vi "Ini files Objects.vi"() -> ()   [LabVIEW 2019]
uses:
  Classes/Parse/ParsePaths/Path.lvclass
  Classes/Parse/Dot/Dot.lvclass
  Classes/Parse/Image/SVGImage.lvclass
  Classes/Parse/Rectangle/Rectangle.lvclass
  Classes/Settings/Dot Settings/Dot Settings.lvclass
  Classes/Settings/Setting Database/Typedefs/PublicEvents--Setting Database.DotsUpdated.ctl
  Classes/Settings/Setting Database/Setting Database.lvclass
  Classes/Settings/Funnel Settings/Funnel Settings.lvclass
  Classes/Settings/Setting Database/Typedefs/PublicEvents--Setting Database.FunnelsUpdated.ctl
  Classes/Settings/Rectangle Settings/Rectangle Settings.lvclass
  Classes/Settings/Setting Database/Typedefs/PublicEvents--Setting Database.RectanglesUpdated.ctl
  Classes/Settings/Path Settings/Path Settings.lvclass
  Classes/Settings/Setting Database/Typedefs/PublicEvents--Setting Database.PathsUpdated.ctl
  Classes/Parse/PathCommands.Moveto/PathCommands.MoveTo.lvclass
  Classes/Parse/PathCommands.CurveTo/PathCommands.CurveTo.lvclass
  Classes/Parse/CSSProperties/CSSProperties.lvclass
  Classes/Parse/Transform.Translate/Transform.Translate.lvclass
  Classes/Parse/PathCommands.LineTo/PathCommands.LineTo.lvclass
  Classes/Parse/Transform.Matrix/Transform.Matrix.lvclass
  Classes/Parse/PathCommands.ClosePath/PathCommands.ClosePath.lvclass
  <vilib>/JKI/JKI SMO/SMO/SMO.lvclass
  <vilib>/JKI/JKI SMO/SMO/Typedefs/SMOState --Enum.ctl
  Classes/Settings/Setting Database/Typedefs/PrivateEvents--Setting Database.Refresh.ctl
  Classes/Archiver/Archivist.lvclass
  <userlib>/_OpenG.lib/lvzip/lvzip.llb/subVI/ZLIB Compress Directory (Path)__ogtk.vi
  C:/Users/Albro/Documents/GitHub/AFM-Lithography/lvsrc/Classes/Settings/ObjectSettings/ObjectSettings.lvclass
  C:/Program Files (x86)/National Instruments/LabVIEW 2019/vi.lib/JKI/JKI SMO/SMO/SMO.lvclass
panel:
  out "GUIDs 2":string[](array[string])
  out "GUIDs":string[](array[string])
  out "Funnels All Updated":bool
  out "Funnels Equal":bool
  out "Rects Equal?":bool
  out "Paths Equal":bool
  out "number of events discarded":u32
  out "Rectangles All Updated":bool
  out "Paths Updated/":bool
  out "error out":errorcluster
  out "Array":string[](array[string])
  out "GUID":string[](array[string])
  # "Why arent GUIDs in Order?"
  # "Close Panel to stop the SMO\n(press the \"X\")"
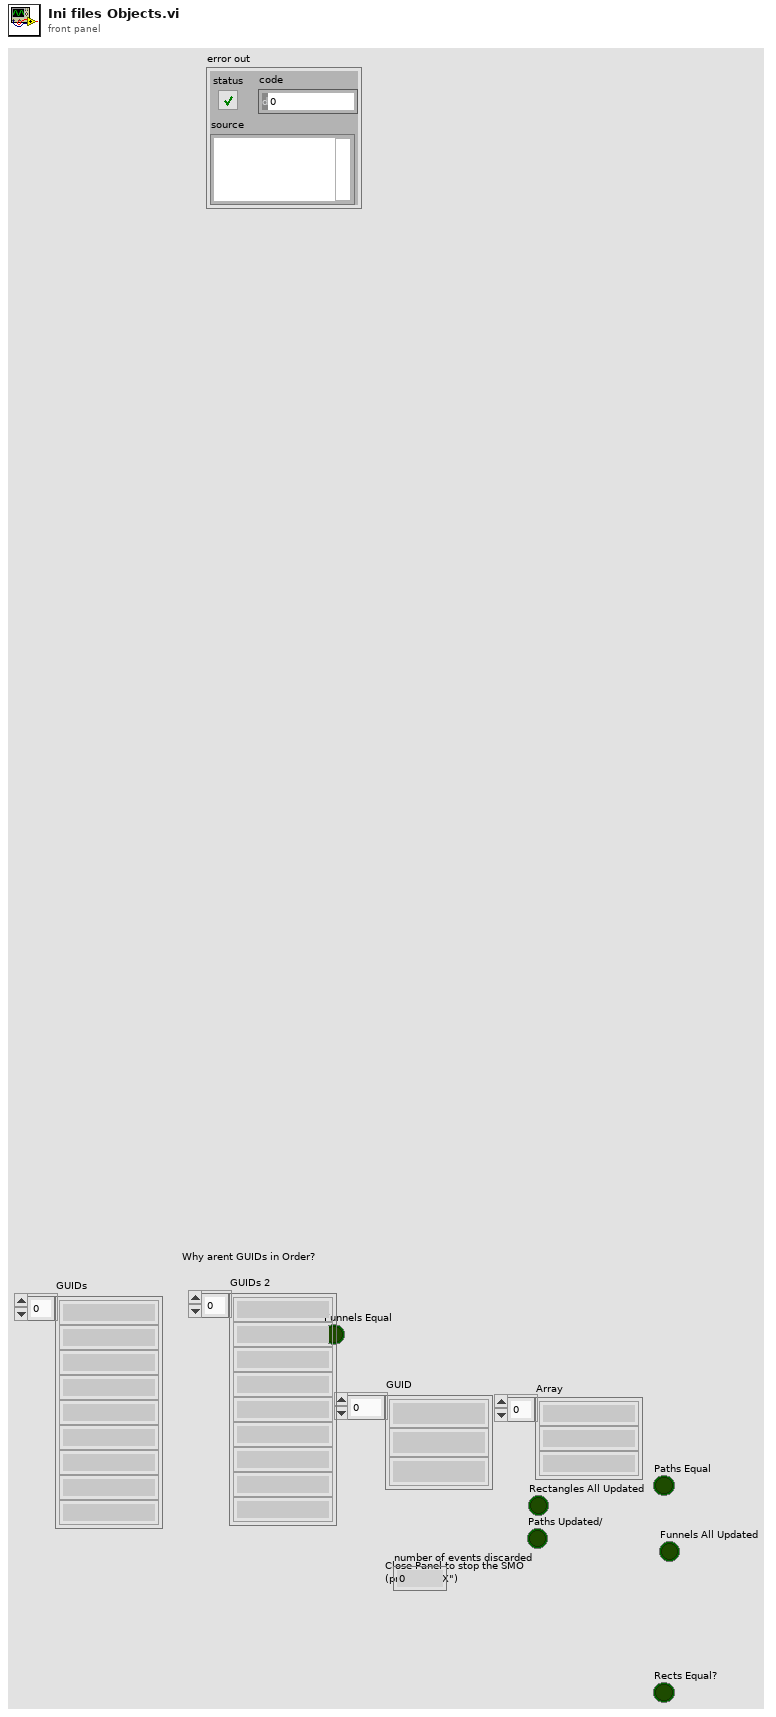
[diagram p1: front panel]
types:
  T1 = typedef "Setting Database.lvclass/PublicEvents--Setting Database.PathsUpdated.ctl" = refnum<class "Path Settings.lvclass">[]
  T2 = typedef "Setting Database.lvclass/PublicEvents--Setting Database.RectanglesUpdated.ctl" = refnum<class "Rectangle Settings.lvclass">[]
  T3 = typedef "Setting Database.lvclass/PublicEvents--Setting Database.FunnelsUpdated.ctl" = refnum<class "Funnel Settings.lvclass">[]
  T4 = typedef "Setting Database.lvclass/PublicEvents--Setting Database.DotsUpdated.ctl" = refnum<class "Dot Settings.lvclass">[]
  T5 = cluster{"Paths":T1, "Rectangles":T2, "Funnels":T3, "Dots":T4}
  T6 = typedef "Setting Database.lvclass/PublicEvents--Cluster.ctl" = cluster{"NewActivePath":refnum<user-event>, "PathsUpdated":refnum<user-event>, "RectanglesUpdated":refnum<user-event>, "NewActiveRectangle":refnum<user-event>, "NewActiveFunnel":refnum<user-event>, "FunnelsUpdated":refnum<user-event>, "NewActiveDot":refnum<user-event>, "DotsUpdated":refnum<user-event>}
  T7 = typedef "SMO.lvclass/Public Events.ctl" = cluster{"Error":refnum<user-event>, "State":refnum<user-event>, "Reserve State":refnum<user-event>}
  T8 = cluster{"Event Registration Refnum":refnum<event-registration>}
  T9 = typedef "Setting Database.lvclass/PrivateEvents--Setting Database.Refresh.ctl" = cluster{"Paths":string[], "Rectangles":string[], "Funnels":string[], "Dots":string[]}
  T10 = cluster{"Settings":cluster{"Paths":T1, "Rectangles":T2, "Funnels":T3, "Dots":T4}, "Data":cluster{"Paths":refnum<class "Path.lvclass">[], "Rectangles":refnum<class "Rectangle.lvclass">[], "SVGImage":refnum<class "SVGImage.lvclass">, "Dots":refnum<class "Dot.lvclass">[], "Funnels":refnum<class "Path.lvclass">[]}}
  T11 = cluster{"paths":string[], "funnels":string[], "rects":string[], "dots":string[]}
  T12 = enum16{"open", "replace", "create", "open or create", "replace or create", "replace or create with confirmation"}
  T13 = typedef "SMO.lvclass/SMOState --Enum.ctl" = enum16{"unknown", "Created", "Started", "Stopped"}
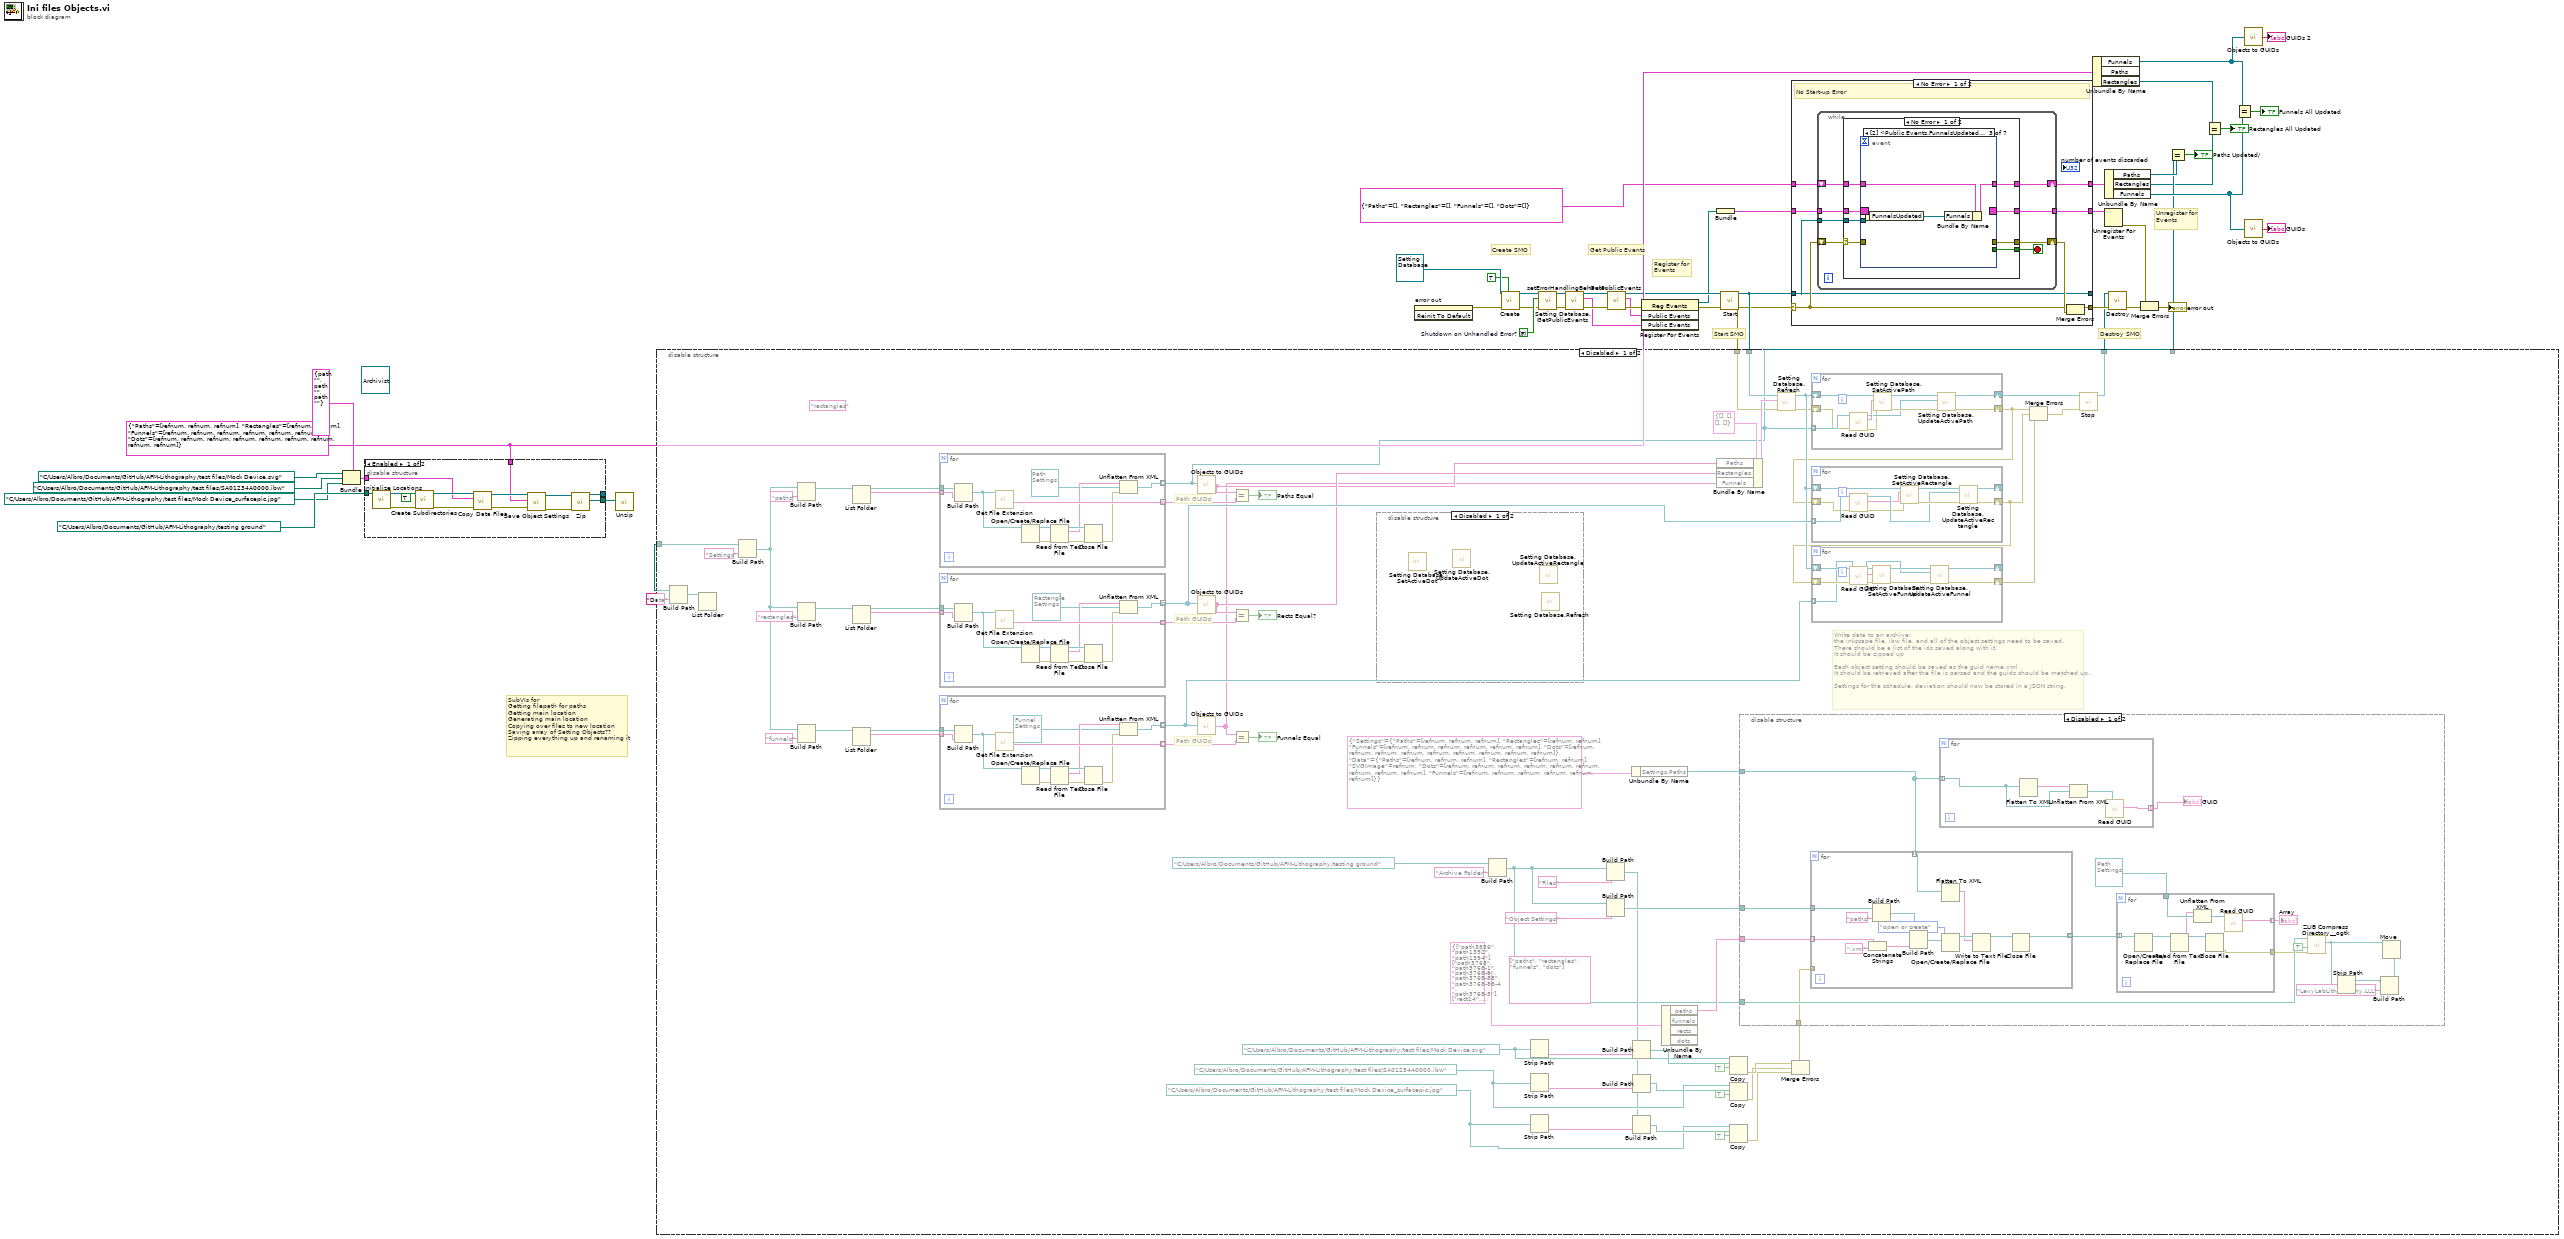
[diagram p0: block diagram]
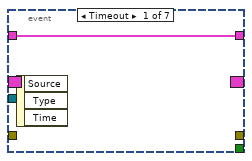
[diagram p2: hidden frame]
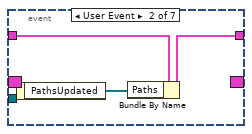
[diagram p3: hidden frame]
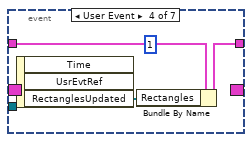
[diagram p4: hidden frame]
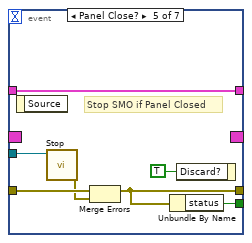
[diagram p5: hidden frame]
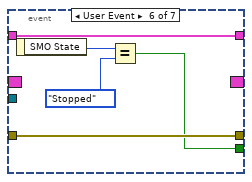
[diagram p6: hidden frame]
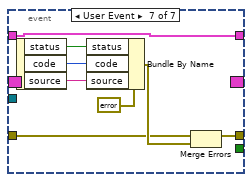
[diagram p7: hidden frame]
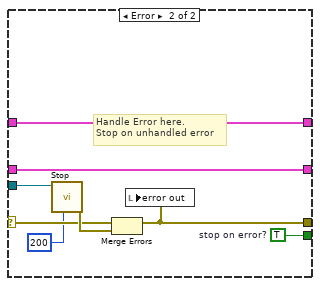
[diagram p8: hidden frame]
diagram:
  w37 = TRUE  # Shutdown on Unhandled Error? (F)
  (unwired) refnum<class "Archivist.lvclass"> refnum ("Archivist.lvclass")
  w42 = T5 {"Paths"=[refnum, refnum, refnum], "Rectangles"=[refnum, refnum], "Funnels"=[refnum, refnum, refnum, refnum, refnum, refnum], "Dots"=[refnum, refnum, refnum, refnum, refnum, refnum, refnum, refnum, refnum]} ("Settings")
  # "Get Public Events"
  # "Start SMO"
  # "Destroy SMO"
  # "Create SMO"
  # "Unregister for Events"
  # "Register for Events"
  # "SubVIs for \nGetting filepath for paths\nGetting main location\nGenerating main location\nCopying over files to new location\nSaving array of Setting Objects??\nZipping everything up and renaming it"
  n1 = Bundle(cluster=cluster{"svg":path, "afm":path, "jpg":path} {"svg"=path "", "afm"=path "", "jpg"=path ""}, "svg"=path "C:/Users/Albro/Documents/GitHub/AFM-Lithography/test files/Mock Device.svg" ("file path"), "afm"=path "C:/Users/Albro/Documents/GitHub/AFM-Lithography/test files/SA01234A0000.ibw" ("file path"), "jpg"=path "C:/Users/Albro/Documents/GitHub/AFM-Lithography/test files/Mock Device_surfacepic.jpg" ("file path")) -> (w41:cluster{"svg":path, "afm":path, "jpg":path})
  n2 = disable-structure shown="Enabled" {
    disable-tunnel: path "C:/Users/Albro/Documents/GitHub/AFM-Lithography/testing ground" ("file path") -> [w60 _]
    disable-tunnel: w42 -> [w56 _]
    disable-tunnel: w41 -> [w55 _]
    disable-tunnel: [w49 _] -> w40
    disable-tunnel: [w48 _] -> _
    frame Enabled {
      (unwired) TRUE ("Archive?")
      n3 = call "Initialize Locations.vi"("Save Location"=w60) -> ("error out"=w54:errorcluster, "Archivist out"=w59:refnum<class "Archivist.lvclass">)  [unwired: 9 in]
      n4 = call "Create Subdirectories.vi"("error in"=w54, "Archivist in"=w59) -> ("error out"=w53:errorcluster, "Archivist out"=w58:refnum<class "Archivist.lvclass">)  [unwired: 8 in]
      n5 = call "Copy Data Files.vi"("error in"=w53, "Data Files"=w55, "Archivist in"=w58) -> ("error out"=w52:errorcluster, "Archivist out"=w57:refnum<class "Archivist.lvclass">)  [unwired: 7 in]
      n6 = call "Save Object Settings.vi"("error in"=w52, "Settings"=w56, "Archivist in"=w57) -> ("error out"=w50:errorcluster, "Archivist out"=w51:refnum<class "Archivist.lvclass">)  [unwired: 7 in]
      n7 = call "Zip.vi"("error in"=w50, "Archivist in"=w51) -> ("archive name out"=w49:path, "Archivist out"=w48:refnum<class "Archivist.lvclass">)  [unwired: 7 in, 1 out]
    }
    frame Disabled {
    }
  }
  n8 = call "Unzip.vi"("Path"=w40) -> ()  [unwired: 9 in, 2 out]
  n9 = invoke on="error out" class="Clust (strict)" method="Reinit To Default"() -> (error out=w38:errorcluster)  [unwired: 3 in, 2 out]
  n10 = call <vilib>:"Create.vi"("Shared Resource (F)"=TRUE, "error in (no error)"=w38, "SMO"=refnum<class "Setting Database.lvclass"> refnum ("Setting Database.lvclass")) -> ("error out"=w36:errorcluster, "SMO out"=w35:refnum<class "Setting Database.lvclass">)  [unwired: 6 in, 1 out]
  n11 = call <vilib>:"setErrorHandlingBehavior.vi"("error in (no error)"=w36, "Shutdown on Unhandled Error? (F)"=w37, "SMO in"=w35) -> ("error out"=w20:errorcluster, "SMO out"=w22:refnum<class "Setting Database.lvclass">)  [unwired: 7 in]
  n12 = call "Setting Database.GetPublicEvents.vi"("error in (no error)"=w20, "Setting Database"=w22) -> ("error out"=w19:errorcluster, "Public Events"=w18:T6, "Setting Database out"=w21:refnum<class "Setting Database.lvclass">)  [unwired: 7 in]
  n13 = call <vilib>:"GetPublicEvents.vi"("error in (no error)"=w19, "SMO"=w21) -> ("error out"=w33:errorcluster, "Public Events"=w32:T7, "SMO out"=w39:refnum<class "Setting Database.lvclass">)  [unwired: 7 in]
  n14 = register-events(error in=w33, w32, w18) -> (reference out=w30:refnum<event-registration>, error out=w31:errorcluster)  [unwired: 1 in]
  n15 = Bundle("Event Registration Refnum"=w30) -> (w26:T8)  [unwired: 1 in]
  n16 = call <vilib>:"Start.vi"("error in (no error)"=w31, "SMO"=w39) -> ("error out"=w11:errorcluster, "SMO out"=w12:refnum<class "Setting Database.lvclass">)  [unwired: 8 in]
  n17 = disable-structure shown="Disabled" {
    disable-tunnel: [w101 _] -> w17
    disable-tunnel: w12 -> [w97 _]
    disable-tunnel: w11 -> [w96 _]
    disable-tunnel: [w62 _] -> w4
    disable-tunnel: [w61 _] -> w1
    frame Disabled {
      (unwired) "rectangles" ("pattern")
      w107 = path "C:/Users/Albro/Documents/GitHub/AFM-Lithography/test files/Mock Device_surfacepic.jpg" ("file path")
      w113 = path "C:/Users/Albro/Documents/GitHub/AFM-Lithography/test files/SA01234A0000.ibw" ("file path")
      w117 = path "C:/Users/Albro/Documents/GitHub/AFM-Lithography/test files/Mock Device.svg" ("file path")
      (unwired) string[] ["paths", "rectangles", "funnels", "dots"]
      # "Path GUIDs"
      # "Path GUIDs"
      # "Path GUIDs"
      # "Write data to an archive:\nthe inkscape file, ibw file, and all of the object settings need to be saved. \nThere should be a list of the ids saved along with it.\nIt should be zipped up\n\nEach object setting should be saved as the guid name.xml\nIt should be retrieved after the file is parsed and the guids should be matched up..\n\nSettings for the schedule, deviation should now be stored in a JSON string."
      n18 = Build Path(base path=w61, name or relative path="Data") -> (appended path=w92:path)
      n19 = List Folder(path=w92) -> ()  [unwired: 3 in, 4 out]
      n20 = Build Path(base path=w61, name or relative path="Settings") -> (appended path=w73:path)
      n21 = Build Path(base path=w73, name or relative path="paths") -> (appended path=w88:path)
      n22 = Build Path(base path=w73, name or relative path="rectangles") -> (appended path=w83:path)
      n23 = Build Path(base path=w73, name or relative path="funnels") -> (appended path=w77:path)
      n24 = List Folder(path=w88) -> (path out=w87:path, filenames=w86:string[])  [unwired: 3 in, 2 out]
      n25 = List Folder(path=w83) -> (path out=w84:path, filenames=w85:string[])  [unwired: 3 in, 2 out]
      n26 = List Folder(path=w77) -> (path out=w78:path, filenames=w79:string[])  [unwired: 3 in, 2 out]
      n27 = for {
        tunnel: w86 -> [w172] mode=indexing
        tunnel: w87 -> [w173]
        tunnel: [w171] -> w90 mode=indexing
        tunnel: [w163] -> w62 mode=indexing
        n28 = Build Path(base path=w173, name or relative path=w172) -> (appended path=w170:path)
        n29 = call <vilib>:"Get File Extension.vi"("file"=w170) -> ("filename without extension"=w171:string)  [unwired: 6 in, 4 out]
        n30 = Open/Create/Replace File(file path (use dialog)=w170) -> (refnum out=w169:refnum<file>, error out=w167:errorcluster)  [unwired: 5 in, 1 out]
        n31 = Read from Text File(file (use dialog)=w169, error in=w167) -> (refnum out=w168:refnum<file>, text=w165:string, error out=w166:errorcluster)  [unwired: 2 in, 1 out]
        n32 = Close File(refnum=w168, error in=w166) -> (error out=w162:errorcluster)  [unwired: 1 out]
        n33 = Unflatten From XML(xml string=w165, type=refnum<class "Path Settings.lvclass"> refnum ("Path Settings.lvclass"), error in (no error)=w162) -> (value=w163:refnum<class "Path Settings.lvclass">)  [unwired: 1 out]
      }
      n34 = for {
        tunnel: w85 -> [w160] mode=indexing
        tunnel: w84 -> [w161]
        tunnel: [w159] -> w81 mode=indexing
        tunnel: [w152] -> w72 mode=indexing
        n35 = Build Path(base path=w161, name or relative path=w160) -> (appended path=w158:path)
        n36 = call <vilib>:"Get File Extension.vi"("file"=w158) -> ("filename without extension"=w159:string)  [unwired: 6 in, 4 out]
        n37 = Open/Create/Replace File(file path (use dialog)=w158) -> (refnum out=w157:refnum<file>, error out=w155:errorcluster)  [unwired: 5 in, 1 out]
        n38 = Read from Text File(file (use dialog)=w157, error in=w155) -> (refnum out=w156:refnum<file>, text=w153:string, error out=w154:errorcluster)  [unwired: 2 in, 1 out]
        n39 = Close File(refnum=w156, error in=w154) -> (error out=w151:errorcluster)  [unwired: 1 out]
        n40 = Unflatten From XML(xml string=w153, type=refnum<class "Rectangle Settings.lvclass"> refnum ("Rectangle Settings.lvclass"), error in (no error)=w151) -> (value=w152:refnum<class "Rectangle Settings.lvclass">)  [unwired: 1 out]
      }
      n41 = for {
        tunnel: w79 -> [w148] mode=indexing
        tunnel: w78 -> [w149]
        tunnel: [w147] -> w75 mode=indexing
        tunnel: [w140] -> w69 mode=indexing
        n42 = Build Path(base path=w149, name or relative path=w148) -> (appended path=w146:path)
        n43 = call <vilib>:"Get File Extension.vi"("file"=w146) -> ("filename without extension"=w147:string)  [unwired: 6 in, 4 out]
        n44 = Open/Create/Replace File(file path (use dialog)=w146) -> (refnum out=w145:refnum<file>, error out=w143:errorcluster)  [unwired: 5 in, 1 out]
        n45 = Read from Text File(file (use dialog)=w145, error in=w143) -> (refnum out=w144:refnum<file>, text=w141:string, error out=w142:errorcluster)  [unwired: 2 in, 1 out]
        n46 = Close File(refnum=w144, error in=w142) -> (error out=w139:errorcluster)  [unwired: 1 out]
        n47 = Unflatten From XML(xml string=w141, type=refnum<class "Funnel Settings.lvclass"> refnum ("Funnel Settings.lvclass"), error in (no error)=w139) -> (value=w140:refnum<class "Funnel Settings.lvclass">)  [unwired: 1 out]
      }
      n48 = call "Objects to GUIDs.vi"("Objects"=w62) -> ("GUIDs"=w70:string[])  [unwired: 3 in, 1 out]
      n49 = call "Objects to GUIDs.vi"("Objects"=w72) -> ("GUIDs"=w71:string[])  [unwired: 3 in, 1 out]
      n50 = call "Objects to GUIDs.vi"("Objects"=w69) -> ("GUIDs"=w68:string[])  [unwired: 3 in, 1 out]
      n51 = Equal?(x=w70, y=w90) -> (x = y?=→"Paths Equal":bool)
      n52 = Equal?(x=w71, y=w81) -> (x = y?=→"Rects Equal?":bool)
      n53 = Equal?(x=w68, y=w75) -> (x = y?=→"Funnels Equal":bool)
      n54 = disable-structure shown="Disabled" {
        frame Disabled {
          n55 = call "Setting Database.SetActiveDot.vi"() -> ()  [unwired: 10 in, 2 out]
          n56 = call "Setting Database.UpdateActiveDot.vi"() -> ()  [unwired: 10 in, 2 out]
          n57 = call "Setting Database.UpdateActiveRectangle.vi"() -> ()  [unwired: 10 in, 2 out]
          n58 = call "Setting Database.Refresh.vi"() -> ()  [unwired: 10 in, 2 out]
        }
        frame Enabled {
        }
      }
      n59 = Build Path(base path=path "C:/Users/Albro/Documents/GitHub/AFM-Lithography/testing ground" ("file path"), name or relative path="Archive Folder") -> (appended path=w106:path)
      n60 = Strip Path(path=w117) -> (name=w119:string)  [unwired: 1 out]
      n61 = Strip Path(path=w113) -> (name=w115:string)  [unwired: 1 out]
      n62 = Strip Path(path=w107) -> (name=w109:string)  [unwired: 1 out]
      n63 = Build Path(base path=w106, name or relative path="Files") -> (appended path=w108:path)
      n64 = Build Path(base path=w106, name or relative path="Object Settings") -> (appended path=w122:path)
      n65 = Unbundle By Name(T10 {"Settings"={"Paths"=[refnum, refnum, refnum], "Rectangles"=[refnum, refnum], "Funnels"=[refnum, refnum, refnum, refnum, refnum, refnum], "Dots"=[refnum, refnum, refnum, refnum, refnum, refnum, refnum, refnum, refnum]}, "Data"={"Paths"=[refnum, refnum, refnum], "Rectangles"=[refnum, refnum], "SVGImage"=refnum, "Dots"=[refnum, refnum, refnum, refnum, refnum, refnum, refnum, refnum, refnum], "Funnels"=[refnum, refnum, refnum, refnum, refnum, refnum]}}) -> ("Settings.Paths"=w120:T1)
      n66 = Build Path(base path=w108, name or relative path=w119) -> (appended path=w118:path)
      n67 = Build Path(base path=w108, name or relative path=w115) -> (appended path=w112:path)
      n68 = Build Path(base path=w108, name or relative path=w109) -> (appended path=w111:path)
      n69 = Unbundle By Name(T11 {"paths"=["path3856", "path1392", "path1394"], "funnels"=["path3768", "path3768-1", "path3768-9", "path3768-88", "path3768-88-4", "path3768-3"], "rects"=["rect14", "rect14-8"], "dots"=["path825", "path825-31", "path825-3", "path825-9", "path825-3-5", "path825-5", "path825-3-4", "path825-9-6", "path825-3-5-2"]} ("IDs")) -> ("paths"=w121:string[])  [unwired: 3 out]
      n70 = Bundle By Name(cluster=T9 {"Paths"=[], "Rectangles"=[], "Funnels"=[], "Dots"=[]} ("Initialize"), "Paths"=w70, "Rectangles"=w71, "Funnels"=w68) -> (w98:T9)
      n71 = Copy(9:TRUE ("overwrite (F)"), 10:w118, 11:w117) -> (0:w105:errorcluster)  [unwired: 2 in, 2 out]
      n72 = Copy(9:TRUE ("overwrite (F)"), 10:w112, 11:w113) -> (0:w104:errorcluster)  [unwired: 2 in, 2 out]
      n73 = Copy(9:TRUE ("overwrite (F)"), 10:w111, 11:w107) -> (0:w103:errorcluster)  [unwired: 2 in, 2 out]
      n74 = call "Setting Database.Refresh.vi"("error in (no error)"=w96, "Initialize"=w98, "Setting Database"=w97) -> ("error out"=w65:errorcluster, "Setting Database out"=w67:refnum<class "Setting Database.lvclass">)  [unwired: 7 in]
      n75 = Merge Errors(w105, w104, w103) -> (w102:errorcluster)
      n76 = disable-structure shown="Disabled" {
        disable-tunnel: w122 -> [w188 _]
        disable-tunnel: w121 -> [w187 _]
        disable-tunnel: w120 -> [w186 _]
        disable-tunnel: w106 -> [w181 _]
        disable-tunnel: w102 -> [w178 _]
        frame Disabled {
          n77 = for {
            tunnel: w188 -> [w213]
            tunnel: w187 -> [w209] mode=indexing
            tunnel: w186 -> [w211] mode=indexing
            tunnel: [w202] -> w183 mode=indexing
            tunnel: w178 -> [_]
            n78 = Concatenate Strings(w209, ".xml" ("string")) -> (w207:string)
            n79 = Build Path(base path=w213, name or relative path="paths") -> (appended path=w210:path)
            n80 = Build Path(base path=w210, name or relative path=w207) -> (appended path=w206:path)
            n81 = Flatten To XML(anything=w211) -> (xml string=w204:string)
            n82 = Open/Create/Replace File(file path (use dialog)=w206, operation (0:open)=T12."open or create") -> (refnum out=w205:refnum<file>)  [unwired: 4 in, 2 out]
            n83 = Write to Text File(file (use dialog)=w205, text=w204) -> (refnum out=w203:refnum<file>)  [unwired: 2 in, 2 out]
            n84 = Close File(refnum=w203) -> (path=w202:path)  [unwired: 1 in, 1 out]
          }
          n85 = for {
            tunnel: w186 -> [w189] mode=indexing
            tunnel: [w190] -> w185 mode=indexing
            n86 = Flatten To XML(anything=w189) -> (xml string=w192:string)
            n87 = Unflatten From XML(xml string=w192, type=w189) -> (value=w191:refnum<class "Path Settings.lvclass">)  [unwired: 1 in, 1 out]
            n88 = call-dynamic "Read GUID.vi"("ObjectSettings in"=w191) -> ("GUID"=w190:string)  [unwired: 8 in, 2 out]
          }
          "GUID" <- w185
          n89 = for {
            tunnel: refnum<class "Path Settings.lvclass"> refnum ("Path Settings.lvclass") -> [w198]
            tunnel: w183 -> [w195] mode=indexing
            tunnel: [w194] -> w182 mode=indexing
            tunnel: [w193] -> w179
            n90 = Open/Create/Replace File(file path (use dialog)=w195) -> (refnum out=w200:refnum<file>)  [unwired: 5 in, 2 out]
            n91 = Read from Text File(file (use dialog)=w200) -> (refnum out=w199:refnum<file>, text=w197:string)  [unwired: 3 in, 2 out]
            n92 = Unflatten From XML(xml string=w197, type=w198) -> (value=w196:refnum<class "Path Settings.lvclass">)  [unwired: 1 in, 1 out]
            n93 = Close File(refnum=w199) -> (error out=w193:errorcluster)  [unwired: 1 in, 1 out]
            n94 = call-dynamic "Read GUID.vi"("ObjectSettings in"=w196) -> ("GUID"=w194:string)  [unwired: 8 in, 2 out]
          }
          "Array" <- w182
          n95 = call-poly <userlib>:"ZLIB Compress Directory__ogtk.vi"("error in (no error)"=w179, "include subdirectories (F)"=TRUE, "root directory (file dialog)"=w181) -> ("archive name out"=w177:path)  [unwired: 6 in, 2 out]
          n96 = Strip Path(path=w177) -> (stripped path=w176:path)  [unwired: 1 out]
          n97 = Build Path(base path=w176, name or relative path="LevyLabLithography.LLL") -> (appended path=w174:path)
          n98 = Move(source path=w177, 10:w174) -> ()  [unwired: 3 in, 3 out]
        }
        frame Enabled {
        }
      }
      n99 = for {
        shift-right: [w231] -> w100
        shift-left: w67 -> [w233]
        shift-right: [w229] -> w64
        shift-left: w65 -> [w225]
        tunnel: w62 -> [w226] mode=indexing
        n100 = call-dynamic "Read GUID.vi"("error in (no error)"=w225, "ObjectSettings in"=w226) -> ("error out"=w224:errorcluster, "GUID"=w228:string, "ObjectSettings out"=w227:refnum<class "Path Settings.lvclass">)  [unwired: 7 in]
        n101 = call "Setting Database.SetActivePath.vi"("error in (no error)"=w224, "SetActivePath"=w228, "Setting Database"=w233) -> ("error out"=w230:errorcluster, "Setting Database out"=w232:refnum<class "Setting Database.lvclass">)  [unwired: 7 in]
        n102 = call "Setting Database.UpdateActivePath.vi"("error in (no error)"=w230, "UpdateCurrentPath"=w227, "Setting Database"=w232) -> ("error out"=w229:errorcluster, "Setting Database"=w231:refnum<class "Setting Database.lvclass">)  [unwired: 7 in]
      }
      n103 = for {
        shift-right: [w221] -> _
        shift-left: w67 -> [w223]
        shift-right: [w220] -> w63
        shift-left: w64 -> [w215]
        tunnel: w72 -> [w216] mode=indexing
        n104 = call-dynamic "Read GUID.vi"("error in (no error)"=w215, "ObjectSettings in"=w216) -> ("error out"=w214:errorcluster, "GUID"=w217:string, "ObjectSettings out"=w218:refnum<class "Rectangle Settings.lvclass">)  [unwired: 7 in]
        n105 = call "Setting Database.SetActiveRectangle.vi"("error in (no error)"=w214, "SetActiveRectangle"=w217, "Setting Database"=w223) -> ("error out"=w219:errorcluster, "Setting Database out"=w222:refnum<class "Setting Database.lvclass">)  [unwired: 7 in]
        n106 = call "Setting Database.UpdateActiveRectangle.vi"("error in (no error)"=w219, "UpdateActiveRectangle"=w218, "Setting Database"=w222) -> ("error out"=w220:errorcluster, "Setting Database"=w221:refnum<class "Setting Database.lvclass">)  [unwired: 7 in]
      }
      n107 = for {
        shift-right: [w133] -> _
        shift-left: w67 -> [w137]
        shift-right: [w134] -> w66
        shift-left: w63 -> [w136]
        tunnel: w69 -> [w129] mode=indexing
        n108 = call-dynamic "Read GUID.vi"("ObjectSettings in"=w129) -> ("GUID"=w131:string, "ObjectSettings out"=w130:refnum<class "Funnel Settings.lvclass">)  [unwired: 8 in, 1 out]
        n109 = call "Setting Database.SetActiveFunnel.vi"("error in (no error)"=w136, "SetActiveFunnel"=w131, "Setting Database"=w137) -> ("error out"=w135:errorcluster, "Setting Database out"=w132:refnum<class "Setting Database.lvclass">)  [unwired: 7 in]
        n110 = call "Setting Database.UpdateActiveFunnel.vi"("error in (no error)"=w135, "UpdateActiveFunnel"=w130, "Setting Database"=w132) -> ("error out"=w134:errorcluster, "Setting Database"=w133:refnum<class "Setting Database.lvclass">)  [unwired: 7 in]
      }
      n111 = Merge Errors(w64, w63, w66) -> (w95:errorcluster)
      n112 = call <vilib>:"Stop.vi"("error in (no error)"=w95, "SMO"=w100) -> ("SMO out"=w101:refnum<class "Setting Database.lvclass">)  [unwired: 8 in, 1 out]
    }
    frame Enabled {
    }
  }
  n113 = case shown="No Error" w11 {
    selector: w11 -> [w237 w298]
    tunnel: [w241 w299] -> w25
    tunnel: w26 -> [w240 w299]
    tunnel: [w238 w298] -> w34
    tunnel: w12 -> [w236 w297]
    tunnel: [w236 w297] -> _
    tunnel: T5 {"Paths"=[], "Rectangles"=[], "Funnels"=[], "Dots"=[]} ("Settings") -> [w235 w296]
    tunnel: [w234 w296] -> w15
    frame No Error {
      # "No Start-up Error"
      n114 = while {
        shift-right: [w248] -> w239
        shift-left: w237 -> [w244]
        tunnel: w240 -> [w247]
        tunnel: [w246] -> w241
        tunnel: w236 -> [w245]
        shift-right: [w242] -> w234
        shift-left: w235 -> [w243]
        stop <- w249 stop-if-true
        n115 = case shown="No Error" w244 {
          selector: w244 -> [w252 w292]
          tunnel: [w257 w295] -> w249
          tunnel: [w256 w289] -> w248
          tunnel: w247 -> [w255 w294]
          tunnel: [w254 w294] -> w246
          tunnel: w245 -> [w253 w291]
          tunnel: w243 -> [w251 w288]
          tunnel: [w250 w288] -> w242
          frame No Error {
            n116 = event shown="[2] <Public Events.FunnelsUpdated>: User Event" {
              selector: w255 -> [_ _ _ _ _ _ _]
              dyn-events: [_ _ _ _ _ _ _] -> w254
              timeout: _ -> [_ _ _ _ _ _ _]
              tunnel: [_ _ _ _ w272 w276 _] -> w257
              tunnel: w253 -> [_ _ _ _ w274 _ _]
              tunnel: [_ _ _ _ w269 w277 w281] -> w256
              tunnel: w252 -> [_ _ _ _ w271 w277 w282]
              tunnel: w251 -> [w258 w260 w263 w265 w268 w275 w280]
              tunnel: [w258 w261 w264 w267 w268 w275 w280] -> w250
              event Timeout {
                n117 = event-data() -> ()  [unwired: 1 in, 3 out]
              }
              event User Event {
                n118 = event-data() -> ("PathsUpdated"=w259:T1)  [unwired: 1 in]
                n119 = Bundle By Name(cluster=w260, "Paths"=w259) -> (w261:T5)
              }
              event User Event {
                n120 = event-data() -> ("FunnelsUpdated"=w262:T3)  [unwired: 1 in]
                n121 = Bundle By Name(cluster=w263, "Funnels"=w262) -> (w264:T5)
              }
              event User Event {
                (unwired) 1 ("keep most recent")
                n122 = event-data() -> ("RectanglesUpdated"=w266:T2)  [unwired: 1 in, 2 out]
                n123 = Bundle By Name(cluster=w265, "Rectangles"=w266) -> (w267:T5)
              }
              event Panel Close? {
                # "Stop SMO if Panel Closed"
                n124 = event-data() -> ()  [unwired: 1 in, 1 out]
                n125 = call <vilib>:"Stop.vi"("SMO"=w274) -> ("error out"=w270:errorcluster)  [unwired: 9 in, 1 out]
                n126 = Merge Errors(w271, w270) -> (w269:errorcluster)
                n127 = Unbundle By Name(w269) -> ("status"=w272:bool)
                n128 = event-data("Discard?"=TRUE ("OK")) -> ()  [unwired: 1 in, 1 out]
              }
              event User Event {
                n129 = event-data() -> ("SMO State"=w279:T13)  [unwired: 1 in]
                n130 = Equal?(x=w279, y=SMOState_--Enum."Stopped") -> (x = y?=w276:bool)
              }
              event User Event {
                n131 = event-data() -> ("status"=w287:bool, "code"=w286:i32, "source"=w285:string)  [unwired: 1 in]
                n132 = Bundle By Name(cluster=errorcluster {"status"=FALSE, "code"=0, "source"=""} ("error out"), "status"=w287, "code"=w286, "source"=w285) -> (w283:errorcluster)
                n133 = Merge Errors(w282, w283) -> (w281:errorcluster)
              }
            }
          }
          frame Error {
            w295 = TRUE  # stop on error?
            # "Handle Error here.\nStop on unhandled error"
            n134 = call <vilib>:"Stop.vi"("timeout in ms (-1)"=200, "SMO"=w291) -> ("error out"=w293:errorcluster)  [unwired: 8 in, 1 out]
            n135 = Merge Errors(w292, w293) -> (w289:errorcluster)
            n136 = local write "error out"(w289) -> ()
          }
        }
      }
      n137 = Merge Errors(w237, w239) -> (w238:errorcluster)
    }
    frame Error {
      # "Error occured before starting the process"
    }
  }
  n138 = Unbundle By Name(w42) -> ("Funnels"=w5:T3, "Rectangles"=w2:T2)  [unwired: 1 out]
  n139 = Unbundle By Name(w15) -> ("Paths"=w14:T1, "Rectangles"=w3:T2, "Funnels"=w8:T3)
  n140 = Unregister For Events(event registration refnum=w25) -> (error out=w27:errorcluster)  [unwired: 1 in]
  n141 = call <vilib>:"Destroy.vi"("error in (no error)"=w34, "SMO"=w17) -> ("error out"=w29:errorcluster)  [unwired: 9 in]
  n142 = Merge Errors(w27, w29) -> (→"error out":errorcluster)
  n143 = Equal?(x=w4, y=w14) -> (x = y?=→"Paths Updated/":bool)
  n144 = Equal?(x=w2, y=w3) -> (x = y?=→"Rectangles All Updated":bool)
  n145 = Equal?(x=w5, y=w8) -> (x = y?=→"Funnels All Updated":bool)
  n146 = call "Objects to GUIDs.vi"("Objects"=w5) -> ("GUIDs"=→"GUIDs 2":string[])  [unwired: 3 in, 1 out]
  n147 = call "Objects to GUIDs.vi"("Objects"=w8) -> ("GUIDs"=→"GUIDs":string[])  [unwired: 3 in, 1 out]
